vi "CmdConsole.Run with Args.vi"(8 "error in (no error)":errorcluster, 9 "Args":string, 10 "StdOutQ":string, 11 "CmdConsole in":refnum<class "CmdConsole.lvclass">) -> (0 "error out":errorcluster, 2 "Running":bool, 3 "CmdConsole out":refnum<class "CmdConsole.lvclass">)   [LabVIEW 2018, in "CmdConsole.lvclass"]
uses:
  CmdConsole.lvclass
  CmdConsole.lvclass/CmdConsole.ctl
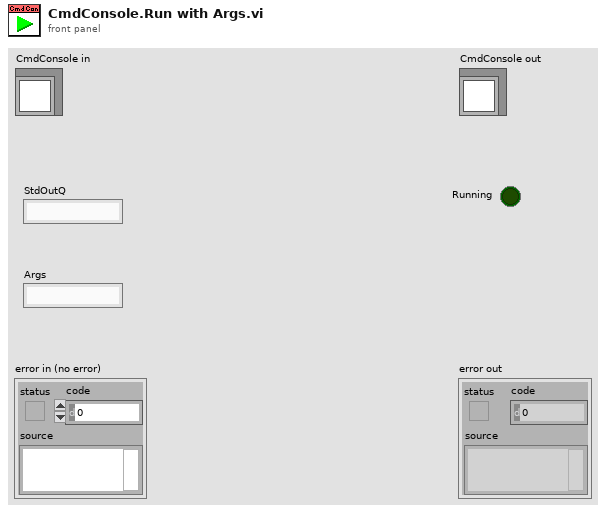
[diagram p1: front panel]
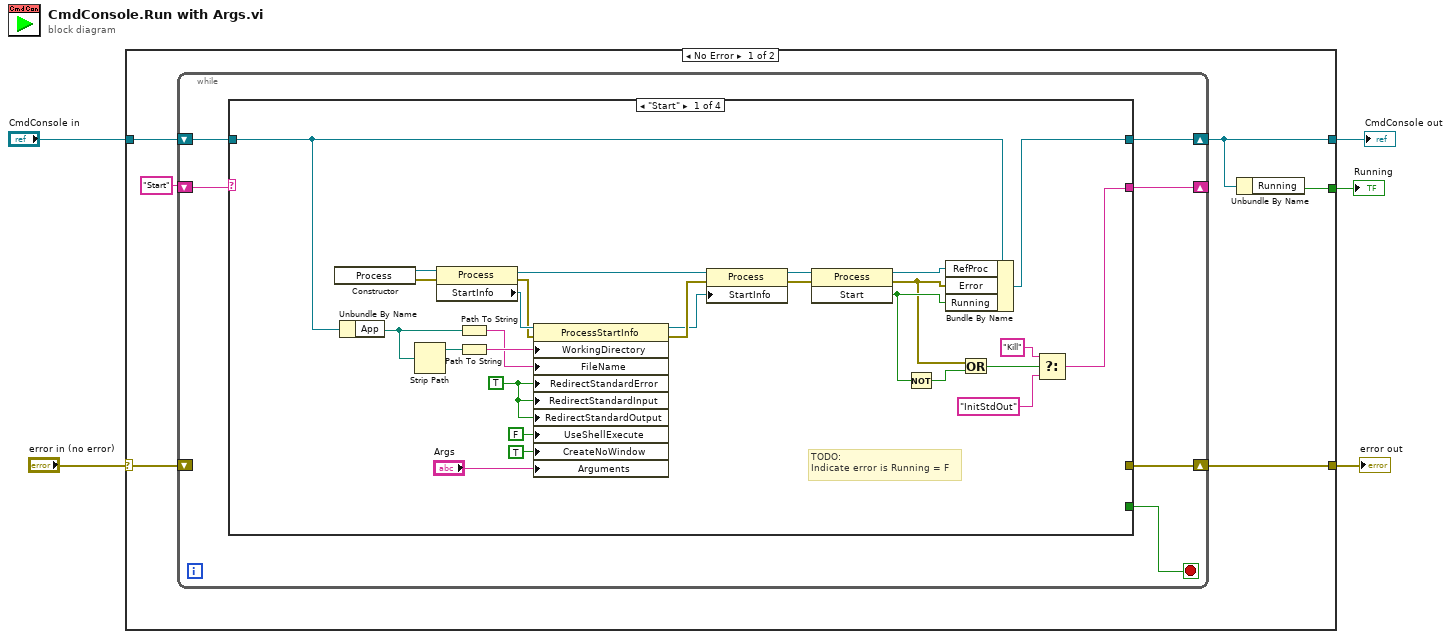
[diagram p0: block diagram]
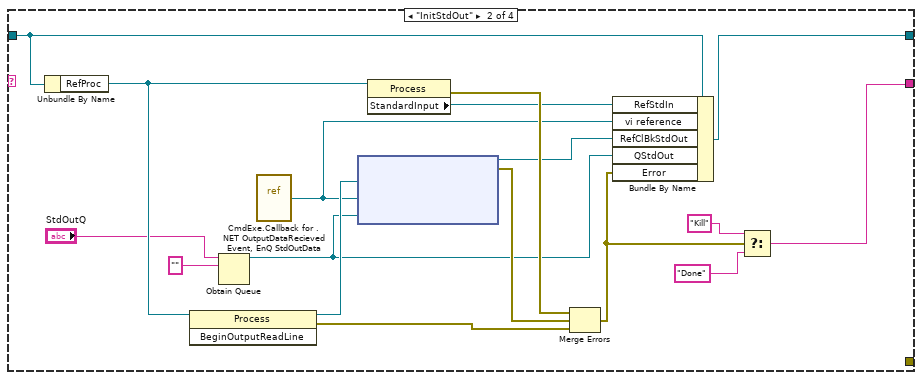
[diagram p2: hidden frame]
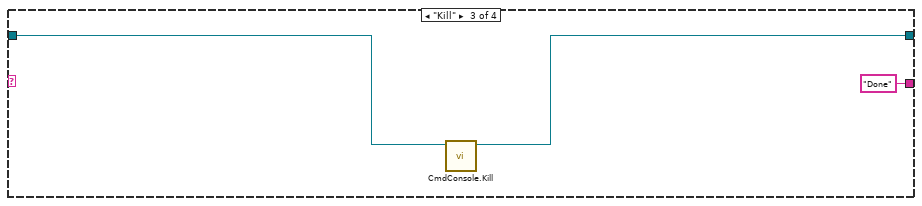
[diagram p3: hidden frame]
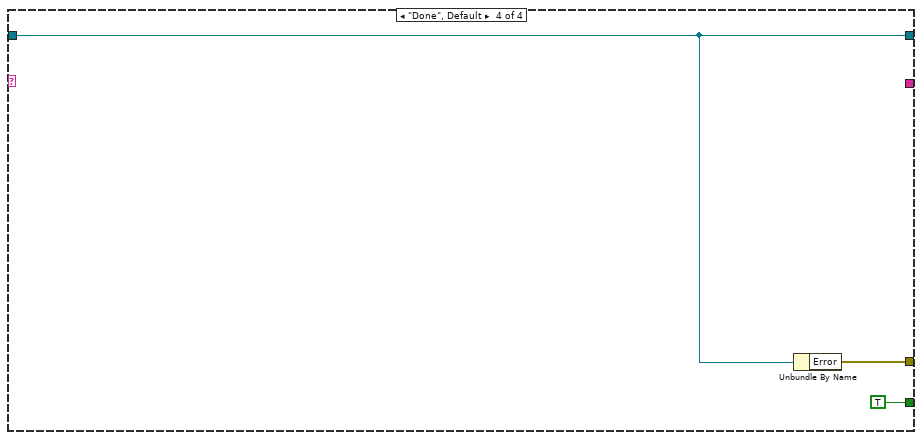
[diagram p4: hidden frame]
diagram:
  n1 = case shown="No Error" "error in (no error)" {
    selector: "error in (no error)" -> [w8 w69]
    tunnel: [w9 w69] -> w4
    tunnel: [w7 w68] -> w2
    tunnel: "CmdConsole in" -> [w11 w68]
    tunnel: [w6 _] -> w1
    frame No Error {
      n2 = while {
        shift-right: [w16] -> w7
        shift-left: w11 -> [w17]
        shift-right: [w14] -> _
        shift-left: "Start" -> [w15]
        shift-right: [w12] -> w9
        shift-left: w8 -> [_]
        stop <- w13 stop-if-true
        n3 = case shown="\"Start\"" w15 {
          tunnel: w17 -> [w44 w55 w64 w66]
          tunnel: [w27 w53 w62 w66] -> w16
          tunnel: [w19 w47 "Done" _] -> w14
          tunnel: [_ _ _ TRUE] -> w13
          tunnel: [_ _ _ w65] -> w12
          frame "Start" {
            w28 = TRUE ("UseShellExecute")
            # "TODO:\nIndicate error is Running = F"
            n4 = constructor class="Process"() -> (reference out=w43:refnum<k24>, error out=w42:errorcluster)  [unwired: 3 in, 1 out]
            n5 = Unbundle By Name(w44) -> ("App"=w29:path)
            n6 = Strip Path(path=w29) -> (stripped path=w32:path)  [unwired: 1 out]
            n7 = property class="Process"(reference=w43, error in=w42) -> (reference out=w35:refnum<k24>, error out=w36:errorcluster, "StartInfo"=w41:refnum<k24>)
            n8 = Path To String(path=w29) -> (string=w30:string)
            n9 = Path To String(path=w32) -> (string=w31:string)
            n10 = property class="ProcessStartInfo"(reference=w41, error in=w36, "WorkingDirectory"=w31, "FileName"=w30, "RedirectStandardError"=w28, "RedirectStandardInput"=w28, "RedirectStandardOutput"=w28, "UseShellExecute"=FALSE, "CreateNoWindow"=TRUE, "Arguments"="Args") -> (reference out=w37:refnum<k24>, error out=w38:errorcluster)
            n11 = property class="Process"(reference=w35, error in=w38, "StartInfo"=w37) -> (reference out=w34:refnum<k24>, error out=w33:errorcluster)
            n12 = invoke class="Process" method="Start"(reference=w34, error in=w33) -> (reference out=w26:refnum<k24>, error out=w23:errorcluster, "Start"=w25:bool)  [unwired: 1 in]
            n13 = Not(x=w25) -> (.not. x?=w24:bool)
            n14 = Bundle By Name(cluster=w44, "RefProc"=w26, "Error"=w23, "Running"=w25) -> (w27:refnum<class "CmdConsole.lvclass">)
            n15 = Or(x=w23, y=w24) -> (x .or. y?=w22:bool)
            n16 = Select(t="Kill", s=w22, f="InitStdOut") -> (s? t:f=w19:string)
          }
          frame "InitStdOut" {
            n17 = Unbundle By Name(w55) -> ("RefProc"=w60:refnum<k24>)
            n18 = invoke class="Process" method="BeginOutputReadLine"(reference=w60) -> (reference out=w61:refnum<k24>, error out=w57:errorcluster)  [unwired: 2 in, 1 out]
            n19 = Obtain Queue(name (unnamed)="StdOutQ", element data type="") -> (queue out=w51:refnum<queue>)  [unwired: 3 in, 2 out]
            n20 = vi-ref "CmdExe.Callback for .NET OutputDataRecieved Event, EnQ StdOutData.vi"() -> ("vi reference"=w45:refnum<vi>)
            n21 = node(w61, w45, w51) -> (w56:refnum<k27>, w58:errorcluster)  [unwired: 2 in]
            n22 = property class="Process"(reference=w60) -> (error out=w59:errorcluster, "StandardInput"=w54:refnum<k24>)  [unwired: 1 in, 1 out]
            n23 = Merge Errors(w59, w58, w57) -> (w50:errorcluster)
            n24 = Bundle By Name(cluster=w55, "RefStdIn"=w54, "vi reference"=w45, "RefClBkStdOut"=w56, "QStdOut"=w51, "Error"=w50) -> (w53:refnum<class "CmdConsole.lvclass">)
            n25 = Select(t="Kill", s=w50, f="Done") -> (s? t:f=w47:string)
          }
          frame "Kill" {
            n26 = call "CmdConsole.Kill.vi"("CmdConsole in"=w64) -> ("CmdConsole out"=w62:refnum<class "CmdConsole.lvclass">)  [unwired: 9 in, 1 out]
          }
          frame "Done", Default {
            n27 = Unbundle By Name(w66) -> ("Error"=w65:errorcluster)
          }
        }
      }
      n28 = Unbundle By Name(w7) -> ("Running"=w6:bool)
    }
    frame Error {
    }
  }
  "error out" <- w4
  "CmdConsole out" <- w2
  "Running" <- w1
